vi "Get Attributes.vi"(8 "error in (no error)":errorcluster, 10 "Only Get DVR":bool, 11 "Web FP In":refnum<class "Web Front Panel.lvclass">) -> (0 "error out":errorcluster, 1 "DataRef":refnum<data-value>, 2 "Data":T1, 3 "Web FP Out":refnum<class "Web Front Panel.lvclass">)   [LabVIEW 2017, in "Front Panel Publisher.lvlib" / "Web Front Panel.lvclass"]
uses:
  Web Front Panel.lvclass
  Protected/Object Attributes.ctl
  Front Panel Objects/Object_class/Object.lvclass
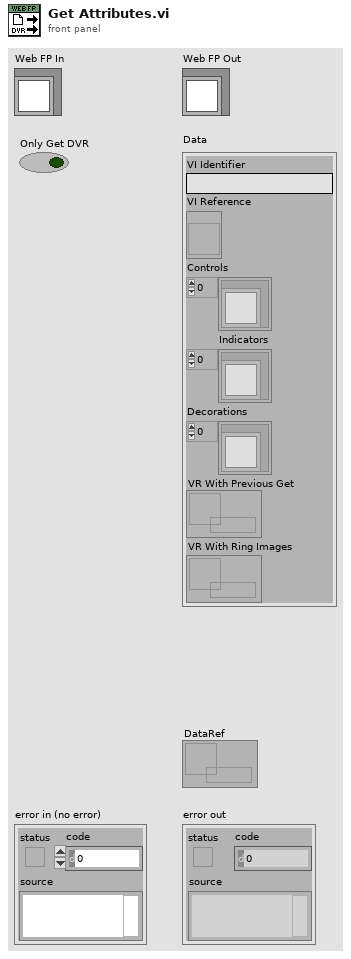
[diagram p1: front panel]
types:
  T1 = typedef "Front Panel Publisher.lvlib/Web Front Panel.lvclass/Object Attributes.ctl" = cluster{"VI Identifier":string, "VI Reference":refnum<vi>, "Controls":refnum<class "Object.lvclass">[], "Indicators":refnum<class "Object.lvclass">[], "Decorations":refnum<class "Object.lvclass">[], "VR With Previous Get":refnum<data-value>, "VR With Ring Images":refnum<data-value>}
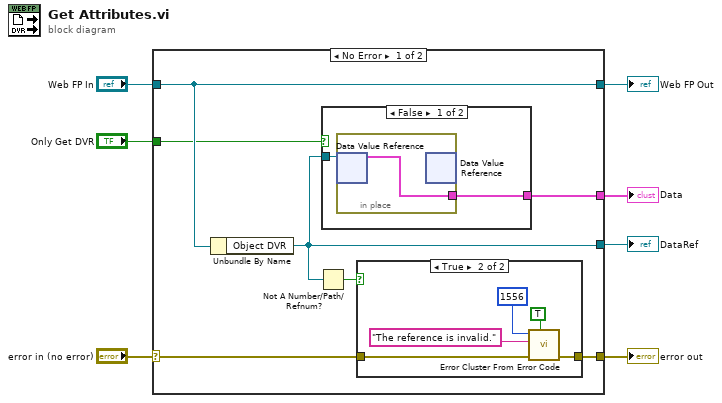
[diagram p0: block diagram]
diagram:
  n1 = case shown="No Error" "error in (no error)" {
    selector: "error in (no error)" -> [w12 w24]
    tunnel: [w10 w24] -> w6
    tunnel: [w14 w25] -> w4
    tunnel: "Web FP In" -> [w14 w25]
    tunnel: [w9 _] -> w3
    tunnel: "Only Get DVR" -> [w13 _]
    tunnel: [w8 _] -> w1
    frame No Error {
      n2 = Unbundle By Name(w14) -> ("Object DVR"=w9:refnum<data-value>)
      n3 = Not A Number/Path/Refnum?(number/path/refnum=w9) -> (NaN/Path/Refnum?=w11:bool)
      n4 = case shown="False" w13 {
        tunnel: w9 -> [w22 _]
        tunnel: [w21 _] -> w8
        frame False {
          n5 = in-place {
            in-place-border: [w23] -> w21
            n6 = in-place-dvr #1(w22) -> (w23:T1)  [unwired: 1 out]
            n7 = in-place-dvr #1() -> ()  [unwired: 1 in, 2 out]
          }
        }
        frame True {
        }
      }
      n8 = case shown="True" w11 {
        tunnel: w12 -> [w15 w17]
        tunnel: [w15 w16] -> w10
        frame False {
        }
        frame True {
          n9 = call <vilib>:"Error Cluster From Error Code.vi"("show call chain? (False)"=TRUE, "error in (no error)"=w17, "error message (\"\")"="The reference is invalid." ("source"), "error code (0)"=1556 ("code")) -> ("error out"=w16:errorcluster)  [unwired: 5 in]
        }
      }
    }
    frame Error {
    }
  }
  "error out" <- w6
  "Web FP Out" <- w4
  "DataRef" <- w3
  "Data" <- w1
